vi "MCL Get Clock Frequency.vi"(9 "handle":i32, 10 "dacfreq":dbl, 11 "adcfreq":dbl) -> (1 "function return":i32, 2 "dacfreq out":dbl, 3 "adcfreq out":dbl)   [LabVIEW 2017, in "Madlib.lvlib"]
doc: "MADLIB_API int MCL_GetClockFrequency(double *adcfreq, double *dacfreq, int handle);"
uses:
  Madlib.lvlib
  Madlib.dll
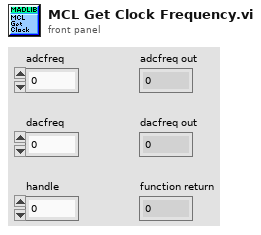
[diagram p1: front panel]
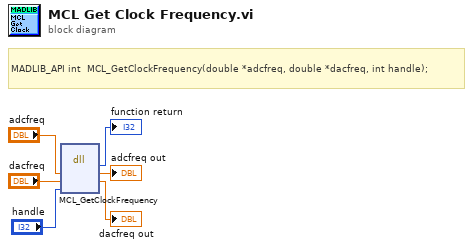
[diagram p0: block diagram]
diagram:
  # "MADLIB_API\tint\t\tMCL_GetClockFrequency(double *adcfreq, double *dacfreq, int handle);"
  n1 = dll-call lib="C:/Users/francesco/dev/pump-probe/Piezo/lvlib/Madlib.*" fn="MCL_GetClockFrequency"("adcfreq"="adcfreq", "dacfreq"="dacfreq", "handle"="handle") -> (→"function return":i32, "adcfreq"=→"adcfreq out":dbl, "dacfreq"=→"dacfreq out":dbl)  [unwired: 4 in, 2 out]
